vi "Save Txt To Xml.vi"() -> ()   [LabVIEW 2016]
uses:
  _vlib/Trial_Info.ctl
  Save Txt To Xml.lvlib
panel:
  in  "SaveToXML":bool
  out "Trials out":T1[](array[typedef]) caption="Таблица событий"
  in  "EEGRead":bool
  out "Progress":i32(slide) caption="Состояние обработки" scale=0.0..14.0
  in  "SampleRateHz":dbl=128.0 caption="Частота дискретизации, Гц"
  in  "EEG file":path caption="Путь к текстовому файлу с ЭЭГ"
  in  "EEG Data Refnum":refnum<data-value>
  in  "Channel Names":string[](array[string])
  in  "Class List":string[](array[string])
  in  "Stop":bool
  # "This VI is a part of BCI Design library, http://www.ru-bci.org \nCopyright © 2020, Sotnikov Peter, All rights reserved. License: GNU GPLv3"
  # "Начало\nпробы"
  # "Конец\nпробы"
  # "Метка\nкласса"
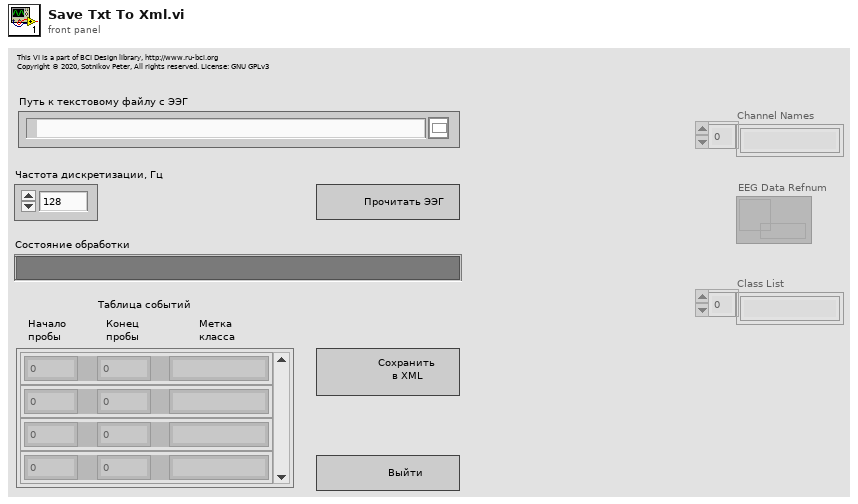
[diagram p1: front panel]
types:
  T1 = typedef "Save Txt To Xml.lvlib/Trial_Info.ctl" = cluster{"Start Position":i32, "End Position":i32, "Class":string}
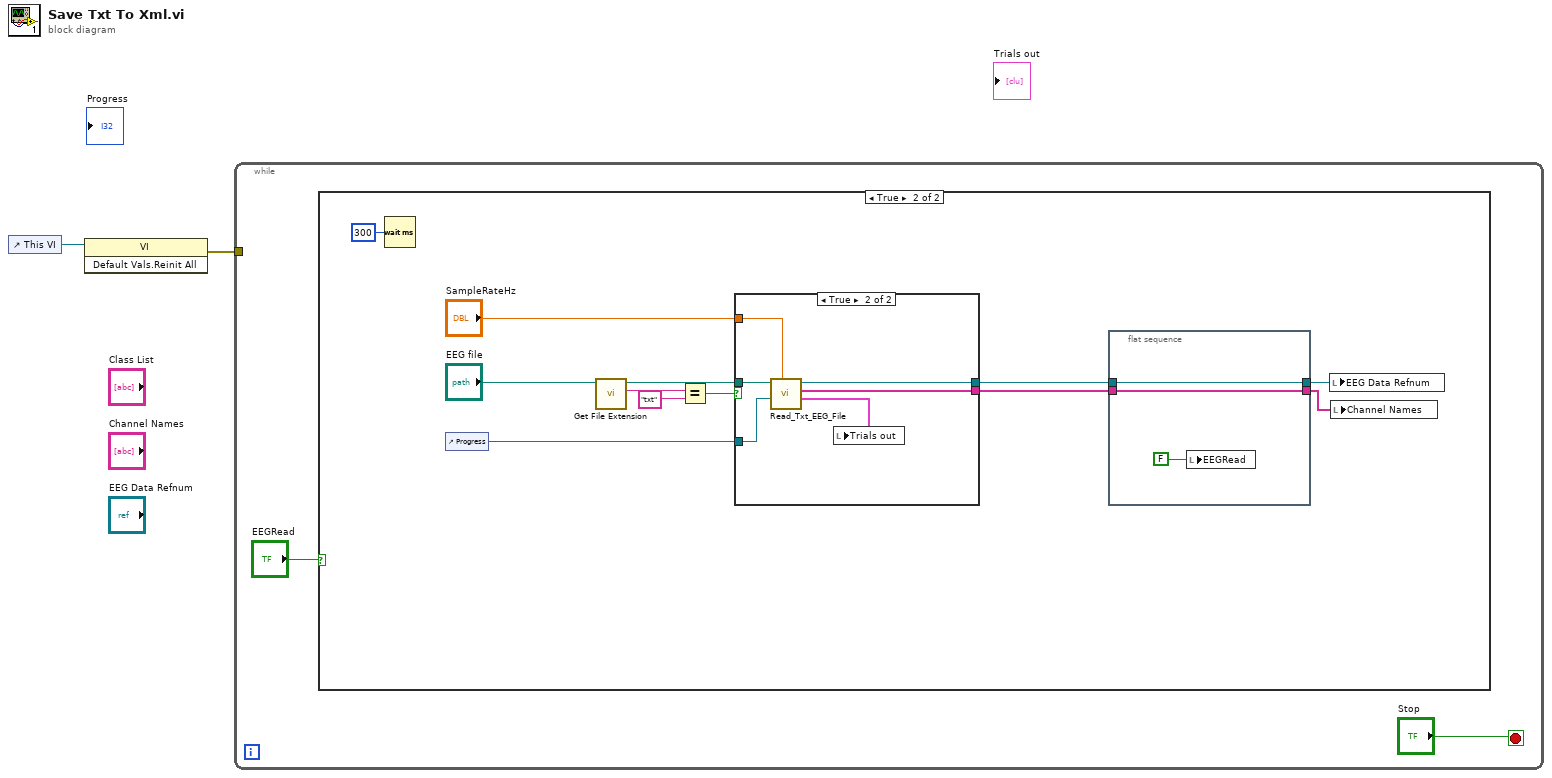
[diagram p0: block diagram]
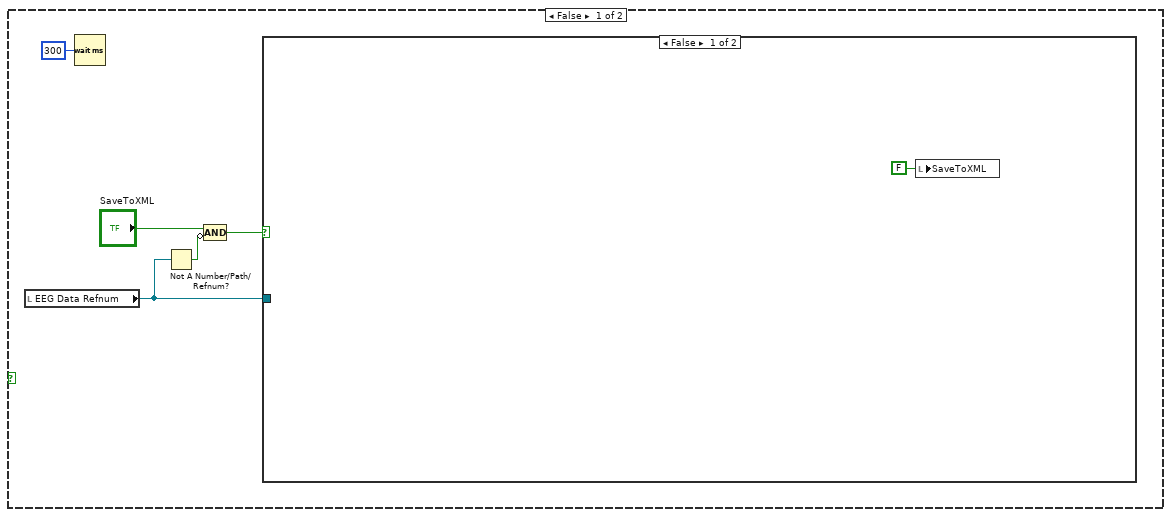
[diagram p2: hidden frame]
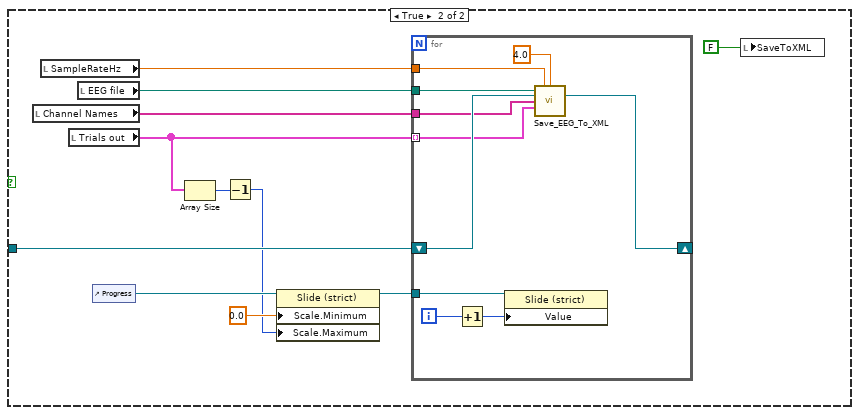
[diagram p3: hidden frame]
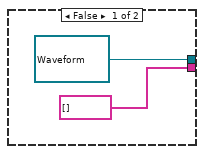
[diagram p4: hidden frame]
diagram:
  n1 = control-ref of="This VI"() -> (w2:refnum<vi>)
  n2 = invoke class="VI" method="Default Vals.Reinit All"(reference=w2) -> (error out=w1:errorcluster)  [unwired: 2 in, 2 out]
  n3 = while {
    tunnel: w1 -> [_]
    stop <- "Stop" stop-if-true
    n4 = case shown="True" "EEGRead" {
      frame False {
        n5 = local read "EEG Data Refnum"() -> (w8:refnum<data-value>)
        n6 = Wait (ms)(milliseconds to wait=u32 300) -> ()  [unwired: 1 out]
        n7 = Not A Number/Path/Refnum?(number/path/refnum=w8) -> (NaN/Path/Refnum?=w7:bool)
        n8 = Compound Arithmetic op=AND("SaveToXML", invert w7) -> (w5:bool)
        n9 = case shown="False" w5 {
          tunnel: w8 -> [_ w13]
          frame False {
            n10 = local write "SaveToXML"(FALSE ("SaveToXML")) -> ()
          }
          frame True {
            n11 = local read "Channel Names"() -> (w18:string[])
            n12 = local read "SampleRateHz"() -> (w20:dbl)
            n13 = local read "Trials out"() -> (w16:T1[])
            n14 = local read "EEG file"() -> (w21:path)
            n15 = control-ref of="Progress"() -> (w17:refnum<vi>)
            n16 = Array Size(array=w16) -> (size(s)=w12:i32)
            n17 = Decrement(x=w12) -> (x-1=w11:i32)
            n18 = property class="Slide (strict)"(reference=w17, "Scale.Minimum"=0.0 ("Scale.Range:Minimum"), "Scale.Maximum"=w11) -> (reference out=w14:refnum<vi>)  [unwired: 1 in, 1 out]
            n19 = for {
              tunnel: w21 -> [w30]
              tunnel: w20 -> [w29]
              shift-right: [w28] -> _
              shift-left: w13 -> [w31]
              tunnel: w16 -> [w25] mode=indexing
              tunnel: w18 -> [w26]
              tunnel: w14 -> [w24]
              i -> [w23]
              n20 = Increment(x=w23) -> (x+1=w22:i32)
              n21 = property class="Slide (strict)"(reference=w24, "Value"=w22) -> ()  [unwired: 1 in, 2 out]
              n22 = call "Save_EEG_To_XML.vi"("Path to EEG File"=w30, "SampleRateHz"=w29, "Epoch Duration"=4.0 ("Event Duration"), "EEG Refnum in"=w31, "ChannelNames in"=w26, "Trial Info"=w25) -> ("EEG Refnum out"=w28:refnum<data-value>)  [unwired: 8 in, 1 out]
            }
            n23 = local write "SaveToXML"(FALSE ("SaveToXML")) -> ()
          }
        }
      }
      frame True {
        n24 = Wait (ms)(milliseconds to wait=u32 300) -> ()  [unwired: 1 out]
        n25 = control-ref of="Progress"() -> (w41:refnum<vi>)
        n26 = call <vilib>:"Get File Extension.vi"("file"="EEG file") -> ("lowercase file extension"=w34:string)  [unwired: 6 in, 4 out]
        n27 = Equal?(x=w34, y="txt") -> (x = y?=w32:bool)
        n28 = case shown="True" w32 {
          tunnel: w41 -> [_ w50]
          tunnel: "SampleRateHz" -> [_ w49]
          tunnel: [refnum<data-value> refnum ("EEG Refnum out") w48] -> w39
          tunnel: [string[] [] ("ChannelNames out") w47] -> w38
          tunnel: "EEG file" -> [_ w46]
          frame False {
          }
          frame True {
            n29 = call "Read_Txt_EEG_File.vi"("SampleRateHz"=w49, "ProgressBarRef"=w50, "EEG file Path in"=w46) -> ("Events out"=w45:T1[], "ChannelNames out"=w47:string[], "EEG Refnum out"=w48:refnum<data-value>)  [unwired: 5 in, 1 out]
            n30 = local write "Trials out"(w45) -> ()
          }
        }
        n31 = flat-sequence {
          tunnel: w39 -> [w52]
          tunnel: [w52] -> w37
          tunnel: w38 -> [w51]
          tunnel: [w51] -> w36
          frame #0 {
            n32 = local write "EEGRead"(FALSE ("Start")) -> ()
          }
        }
        n33 = local write "EEG Data Refnum"(w37) -> ()
        n34 = local write "Channel Names"(w36) -> ()
      }
    }
  }
